vi "Task1.vi"() -> ()   [LabVIEW 2022 SP3]
panel:
  out "Noise Voltage (V)":dbl
  in  "Bandwidth (Hz)":dbl
  in  "Resistance (Ohm)":dbl
  in  "Temperature (K)":dbl
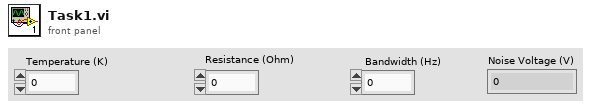
[diagram p1: front panel]
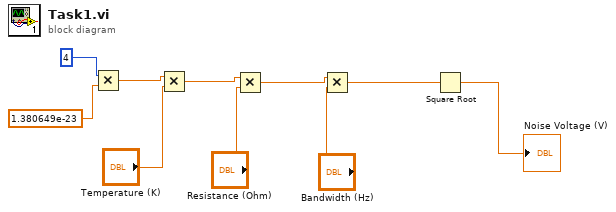
[diagram p0: block diagram]
diagram:
  n1 = Multiply(x=4, y=1.380649e-23) -> (x*y=w7:dbl)
  n2 = Multiply(x=w7, y="Temperature (K)") -> (x*y=w5:dbl)
  n3 = Multiply(x=w5, y="Resistance (Ohm)") -> (x*y=w3:dbl)
  n4 = Multiply(x=w3, y="Bandwidth (Hz)") -> (x*y=w2:dbl)
  n5 = Square Root(x=w2) -> (sqrt(x)=→"Noise Voltage (V)":dbl)
